vi "Quit.vi"(8 "error in (no error)":errorcluster, 11 "AB_UI_Frmwk_Installer in":refnum<class "AB_UI_Frmwk_Installer.lvclass">) -> (0 "error out":errorcluster, 3 "AB_UI_Frmwk_Installer out":refnum<class "AB_UI_Frmwk_Installer.lvclass">)   [LabVIEW 2020, in "AB_UI_Frmwk_Installer.lvclass"]
uses:
  <vilib>/AppBuilder/IB_Classes/Installer/UI/AB_UI_Frmwk_Installer.lvclass
  <vilib>/AppBuilder/IB_Classes/Installer/UI/AB_UI_Frmwk_Installer.lvclass/AB_UI_Frmwk_Installer.ctl
  AppLibs/distkit/MDF/NI_MDF.lvlib
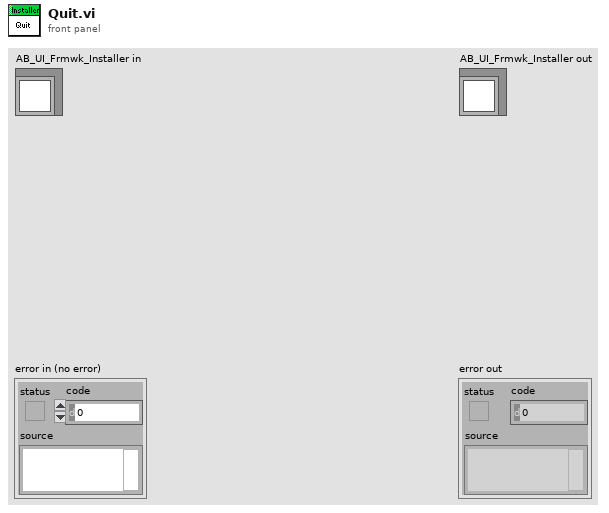
[diagram p1: front panel]
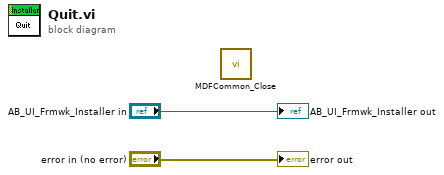
[diagram p0: block diagram]
diagram:
  n1 = call "MDFCommon_Close.vi"() -> ()  [unwired: 1 in, 11 out]
  "error out" <- "error in (no error)"
  "AB_UI_Frmwk_Installer out" <- "AB_UI_Frmwk_Installer in"
